vi "set register bits.vi"(0 "address":u8, 3 "register bits":bool[](array[boolean])=[FALSE, FALSE, FALSE, FALSE, FALSE, FALSE, FALSE, FALSE]) -> (6 "address / value":u8[](array[numeric]))   [LabVIEW 2013]
doc: "Set the bits of an 8-bit I2C register with values specified in a Boolean array. The subVI accepts an 8-element Boolean array (with element 0 taken as the most-significant bit) and an I2C register address and creates a two-element byte array (address followed by register value) for use by the NI myRIO I2C subVIs."
panel:
  # "Set Register Bits"
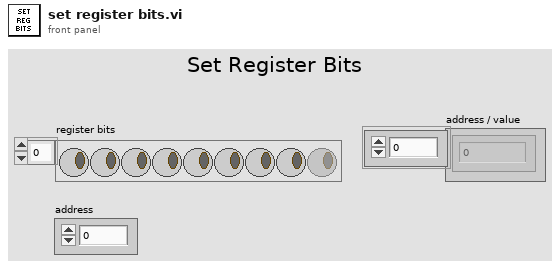
[diagram p1: front panel]
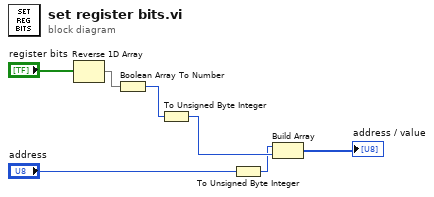
[diagram p0: block diagram]
diagram:
  n1 = Reverse 1D Array(array="register bits") -> (reversed array=w3:bool[])
  n2 = Boolean Array To Number(Boolean array=w3) -> (number=w4:u32)
  n3 = To Unsigned Byte Integer(number=w4) -> (unsigned 8bit integer=w7:u8)
  n4 = To Unsigned Byte Integer(number="address") -> (unsigned 8bit integer=w6:u8)
  n5 = Build Array "Build Array"(w6, w7) -> (→"address / value":u8[])
